vi "Continuous Acquisition from PSD software norm.vi"() -> ()   [LabVIEW 2010]
doc: "I. Description:\nThis example demonstrates how to acquire a continuous amount of data (Waveform) using the DAQ device's internal clock.\n\nII. Instructions for Running:\n1. Create an analog input voltage channel.\n2. Set the rate for the sample clock. Additionally, define the sample mode to be continuous.\n3. Call the Start VI to start the acquisition.\n4. Read the waveform data in a loop until the user hits the stop button or an error occurs.\nNote: This example reads data from one or more channels and returns an array of data. Use the Index Array function to access an individual channel of data.\n5. Call the Clear Task VI to clear the Task.\n6. Use the popup dialog box to display an error if any.\n\nIV. I/O Connections Overview:\nMake sure your signal input terminal matches the Physical Channel I/O Control. For further connection information, refer to your hardware reference manual."
uses:
  <vilib>/Utility/error.llb/DialogType.ctl
  <vilib>/DAQmx/read.llb/DAQmx Read (Analog 2D DBL NChan NSamp).vi
  <vilib>/DAQmx/create/channels.llb/DAQmx Create Channel (AI-Voltage-Basic).vi
  <vilib>/DAQmx/configure/timing.llb/DAQmx Timing (Sample Clock).vi
  <vilib>/daqmx/miscellaneous.llb/DAQmx Fill In Error Info.vi
panel:
  out "XY Graph (Va diff vs Vc diff)":T1(graph)
  out "Raw Signals":dbl[][](graph)
  out "XY Graph (Va vs Vc)":T1(graph)
  out "Normalized Signals":dbl[][](graph)
  in  "Samples to Read":i32=1000
  in  "stop":bool
  in  "Sample Rate":dbl=10000.0 caption="Sample Rate (Hz)" format="%.1f"
  # "Note:\n\nPCI-6251 board\nmax sampling rate\nis 1MS/s in\nscanning mode.\n\nThis VI scans\n 5 channels\nso 200kS/s \nis the max."
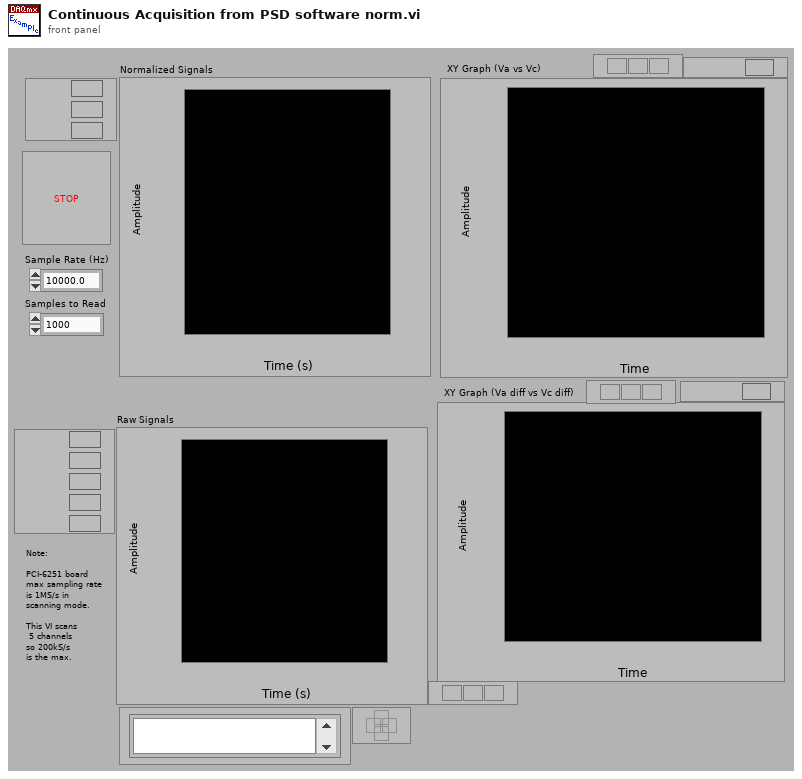
[diagram p1: front panel]
types:
  T1 = cluster{"Normalized positions\n(Vc, Va)":dbl[], "Normalized positions\n(Vc, Va)":dbl[]}
  T2 = typedef "DialogType.ctl" = u16
  T3 = cluster{"Normalized positions\n(Vc, Va, sum)":dbl[], "Normalized positions\n(Vc, Va, sum)":dbl[]}
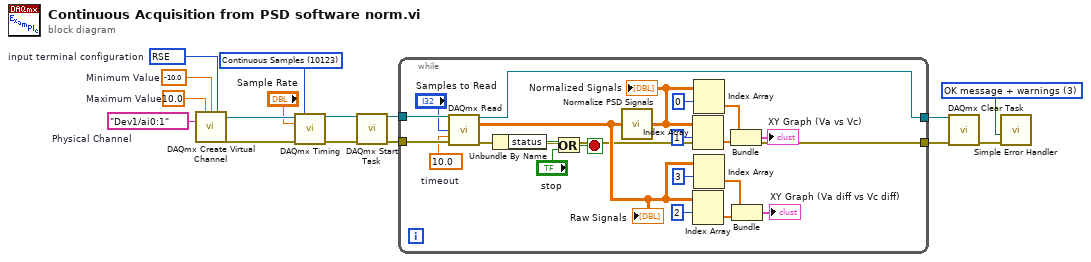
[diagram p0: block diagram]
diagram:
  w8 = tag "Dev1/ai0:1"  # Physical Channel
  w15 = 10.0  # Maximum Value
  w16 = -10.0  # Minimum Value
  w1 = 10083 items=["default"=-1, "RSE"=10083, "NRSE"=10078, "Differential"=10106, "Pseudodifferential"=12529]  # input terminal configuration
  w2 = T2 3 items=["no dialog", "OK message", "continue or stop message", "OK message + warnings", "continue/stop + warnings"] ("type of dialog (OK msg:1)")
  w7 = 10123 items=["Finite Samples"=10178, "Continuous Samples"=10123] ("sample mode")
  n1 = call-poly <vilib>:"DAQmx Create Virtual Channel.vi"("maximum value"=w15, "minimum value"=w16, "input terminal configuration"=w1, "physical channels"=w8) -> ("task out"=w11:refnum<k21>, "error out"=w14:errorcluster)  [unwired: 10 in]
  n2 = call-poly <vilib>:"DAQmx Timing.vi"("task/channels in"=w11, "sample mode"=w7, "rate"="Sample Rate", "error in"=w14) -> ("task out"=w6:refnum<k21>, "error out"=w5:errorcluster)  [unwired: 10 in]
  n3 = call <vilib>:"DAQmx Start Task.vi"("task/channels in"=w6, "error in"=w5) -> ("task out"=w10:refnum<k21>, "error out"=w13:errorcluster)  [unwired: 12 in]
  n4 = while {
    tunnel: w13 -> [w37]
    tunnel: w10 -> [w36]
    tunnel: [w18] -> w9
    tunnel: [w19] -> w4
    stop <- w34 stop-if-true
    w32 = 10.0  # timeout
    n5 = call-poly <vilib>:"DAQmx Read.vi"("task/channels in"=w36, "number of samples per channel"="Samples to Read", "timeout"=w32, "error in"=w37) -> ("task out"=w18:refnum<k21>, "data"=w23:dbl[][], "error out"=w19:errorcluster)  [unwired: 9 in]
    "Raw Signals" <- w23
    n6 = Unbundle By Name(w19) -> ("status"=w35:bool)
    n7 = Or(x=w35, y="stop") -> (x .or. y?=w34:bool)
    n8 = call "Normalize PSD Signals.vi"("Raw PSD voltages\n(Vc sum, Va sum, Va diff, Vc diff)"=w23) -> ("Normalized positions\n(Vc, Va, sum)"=w17:dbl[][])
    "Normalized Signals" <- w17
    n9 = Index Array(array=w17, index (row)=1) -> (element=w28:dbl[])  [unwired: 1 in]
    n10 = Index Array(array=w23, index (row)=2) -> (element=w20:dbl[])  [unwired: 1 in]
    n11 = Index Array(array=w17, index (row)=0) -> (element=w29:dbl[])  [unwired: 1 in]
    n12 = Index Array(array=w23, index (row)=3) -> (element=w21:dbl[])  [unwired: 1 in]
    n13 = Bundle("Normalized positions\n(Vc, Va, sum)"=w29, "Normalized positions\n(Vc, Va, sum)"=w28) -> (→"XY Graph (Va vs Vc)":T3)  [unwired: 1 in]
    n14 = Bundle("data"=w21, "data"=w20) -> (→"XY Graph (Va diff vs Vc diff)":cluster{"data":dbl[], "data":dbl[]})  [unwired: 1 in]
  }
  n15 = call <vilib>:"DAQmx Clear Task.vi"("task in"=w9, "error in"=w4) -> ("error out"=w12:errorcluster)  [unwired: 13 in]
  n16 = call <vilib>:"Simple Error Handler.vi"("type of dialog (OK msg:1)"=w2, "error in (no error)"=w12) -> ()  [unwired: 3 in, 5 out]
